vi "Bitwise OR (Greyscale with Mask).vi"(6 "Mask in":T1, 8 "error in (no error)":errorcluster, 9 "Greyscale Image Destination in":T1, 10 "Greyscale Image B in":T1, 11 "Greyscale Image A in":T1) -> (0 "error out":errorcluster, 3 "Greyscale Image Destination":T1)   [LabVIEW 2020, in "image.lvlib"]
doc: "Compute the bitwise OR of the pixels in the A and B input images with a mask."
uses:
  image.lvlib
  Greyscale Image.ctl
  BitwiseOperation.ctl
  0e84d7da-7af3-4d73-801a-9d94e7981347.vi
  <vilib>/Utility/error.llb/Error Cluster From Error Code.vi
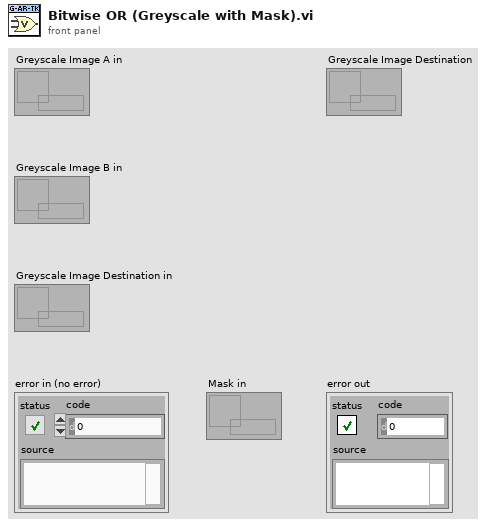
[diagram p1: front panel]
types:
  T1 = typedef "image.lvlib/Greyscale Image.ctl" = refnum<data-value>
  T2 = typedef "image.lvlib/BitwiseOperation.ctl" = enum8{"OR", "AND", "XOR"}
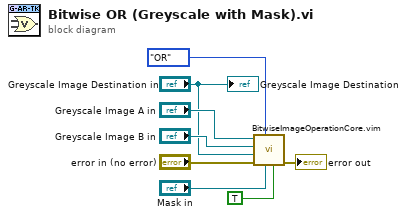
[diagram p0: block diagram]
diagram:
  n1 = call "BitwiseImageOperationCore.vim"("HasMask"=TRUE, "Mask"="Mask in", "BitwiseOperation"=BitwiseOperation."OR", "error in (no error)"="error in (no error)", "Destination Image"="Greyscale Image Destination in", "Image B"="Greyscale Image B in", "Image A"="Greyscale Image A in") -> ("error out"=→"error out":errorcluster)  [unwired: 4 in]
  "Greyscale Image Destination" <- "Greyscale Image Destination in"
